vi "create.vi"(0 "MDILCFactory in":refnum<class "MDILCFactory.lvclass">, 5 "MDSettings":T3, 7 "ILCTimings":T2, 9 "MDTimings":T1, 11 "error in (no error)":errorcluster) -> (4 "MDILCFactory out":refnum<class "MDILCFactory.lvclass">, 6 "MDILC":refnum<class "MDILC.lvclass">, 15 "error out":errorcluster)   [LabVIEW 2016, in "RTMDILC.lvlib" / "MDILCFactory.lvclass"]
uses:
  MDILCFactory.lvclass
  DataTypes/MDSettings.ctl
  Common_RT_ILC/DataTypes/ILCSettings.ctl
  MDILC/MDILC.lvclass
  D:/Code/Common_RT_ILC/ILC/ILC.lvclass
  Common_RT_ILC/DataTypes/ILCTimings.ctl
  DataTypes/MDTimings.ctl
  Common_RT_ILC/ILCFactory/ILCFactory.lvclass
  DataTypes/MDData.ctl
  DataTypes/MDConstants.ctl
  DataTypes/MDTelemetry.ctl
  DataTypes/MDResponses.ctl
  Common_RT_Modbus/DataTypes/ExceptionCodes.ctl
  MDILC/MDILC.lvclass/MDILC.ctl
  RTMDILC.lvlib
  Common_RT_Modbus/RTModbus.lvlib
  Common_RT_ILC/RTILC.lvlib
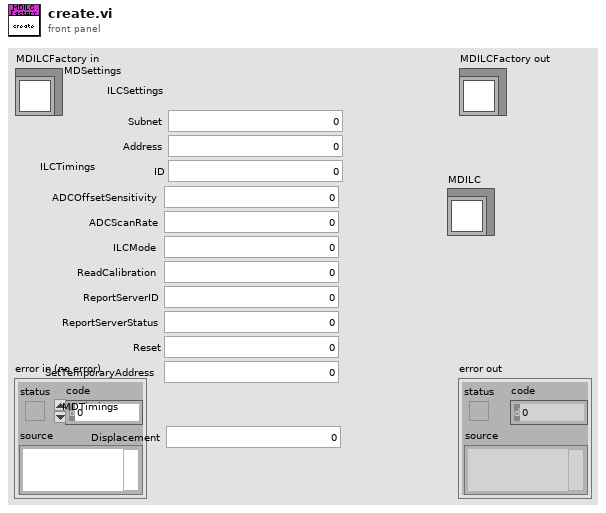
[diagram p1: front panel]
types:
  T1 = typedef "RTMDILC.lvlib/MDTimings.ctl" = cluster{"Displacement":u32}
  T2 = typedef "RTILC.lvlib/ILCTimings.ctl" = cluster{"ADCOffsetSensitivity":u32, "ADCScanRate":u32, "ILCMode":u32, "ReadCalibration":u32, "ReportServerID":u32, "ReportServerStatus":u32, "Reset":u32, "SetTemporaryAddress":u32}
  T3 = typedef "RTMDILC.lvlib/MDSettings.ctl" = cluster{"ILCSettings":T4, "ID":i16}
  T4 = typedef "RTILC.lvlib/ILCSettings.ctl" = cluster{"Subnet":u8, "Address":u8}
  T5 = typedef "RTMDILC.lvlib/MDData.ctl" = cluster{"Constants":T6, "Telemetry":T7, "Responses":T8, "Timings":T1}
  T6 = typedef "RTMDILC.lvlib/MDConstants.ctl" = cluster{"ID":i16}
  T7 = typedef "RTMDILC.lvlib/MDTelemetry.ctl" = cluster{"Displacement":sgl[]}
  T8 = typedef "RTMDILC.lvlib/MDResponses.ctl" = cluster{"Displacement":T9}
  T9 = typedef "RTModbus.lvlib/ExceptionCodes.ctl" = u16
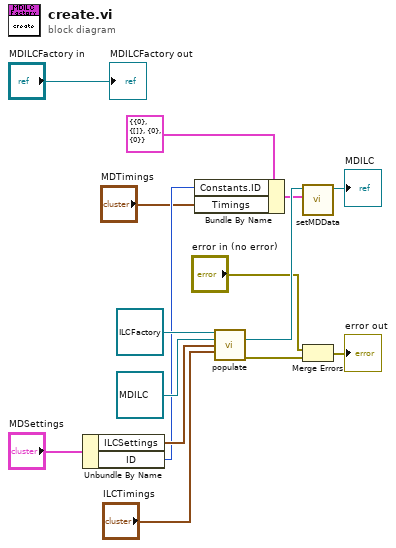
[diagram p0: block diagram]
diagram:
  n1 = Unbundle By Name("MDSettings") -> ("ILCSettings"=w14:T4, "ID"=w9:i16)
  n2 = Bundle By Name(cluster=T5 {"Constants"={"ID"=0}, "Telemetry"={"Displacement"=[]}, "Responses"={"Displacement"=0}, "Timings"={"Displacement"=0}} ("MTData"), "Constants.ID"=w9, "Timings"="MDTimings") -> (w8:T5)
  n3 = call "populate.vi"("ILCFactory in"=refnum<class "ILCFactory.lvclass"> refnum ("RTILC.lvlib:ILCFactory.lvclass"), "ILC in"=refnum<class "MDILC.lvclass"> refnum ("RTMTILC.lvlib:MTILC.lvclass"), "Settings"=w14, "Timings"="ILCTimings") -> ("ILC out"=w11:refnum<class "MDILC.lvclass">, "error out"=w6:errorcluster)  [unwired: 9 in, 1 out]
  n4 = call "setMDData.vi"("MDData"=w8, "MDILC in"=w11) -> ("MDILC out"=→"MDILC":refnum<class "MDILC.lvclass">)  [unwired: 9 in]
  n5 = Merge Errors("error in (no error)", w6) -> (→"error out":errorcluster)
  "MDILCFactory out" <- "MDILCFactory in"
